vi "PID_old.vi"(6 "(t-1)in":dbl, 8 "error in":errorcluster, 9 "Low_Limit (0)":dbl, 10 "Up_Limit (40)":dbl, 11 "Ain":dbl=1.543879594670716 format="%0.2f") -> (0 "error out":errorcluster, 3 "Aout":dbl, 4 "(t-1)out":dbl)   [LabVIEW 2016]
doc: "Подпрограмма основана на непонятной\nмодели физического процесса и его\nреакции на ПИД регулирование.\nВ программу введена для сопоставления\nс предыдущими результатами."
panel:
  # "Подпрограмма основана на непонятной\nмодели физического процесса и его\nреакции на ПИД регулирование.\nВ программу введена для сопоставления\nс предыдущими результатами."
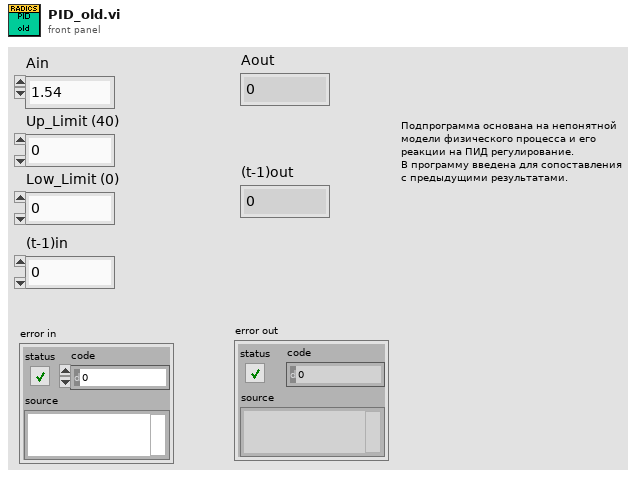
[diagram p1: front panel]
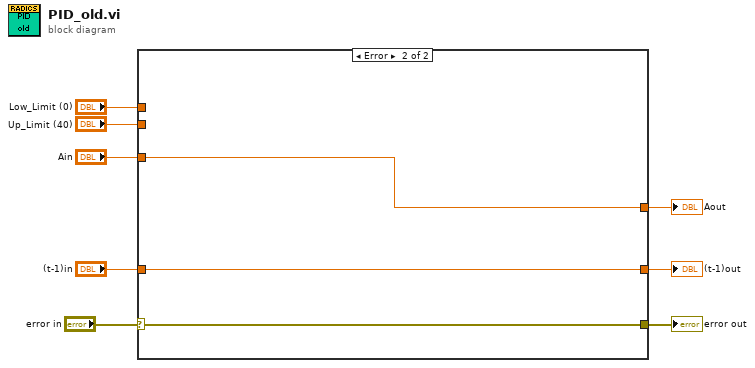
[diagram p0: block diagram]
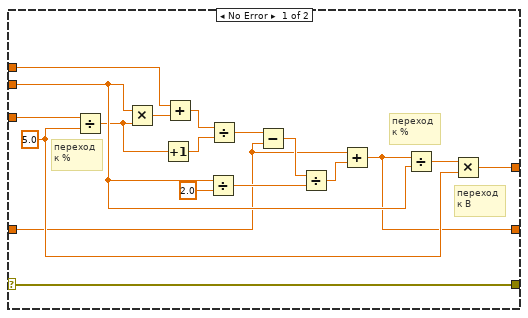
[diagram p2: hidden frame]
diagram:
  n1 = case shown="Error" "error in" {
    selector: "error in" -> [w11 w29]
    tunnel: [w26 w28] -> w8
    tunnel: "Up_Limit (40)" -> [w23 _]
    tunnel: "Low_Limit (0)" -> [w14 _]
    tunnel: "Ain" -> [w12 w28]
    tunnel: [w11 w29] -> w3
    tunnel: "(t-1)in" -> [w10 w27]
    tunnel: [w9 w27] -> w1
    frame No Error {
      w25 = 5.0 ("y")
      # "переход \nк В"
      # "переход \nк %"
      # "переход \nк %"
      n2 = Divide(x=w12, y=w25) -> (x/y=w15:dbl)
      n3 = Multiply(x=w23, y=w15) -> (x*y=w13:dbl)
      n4 = Increment(x=w15) -> (x+1=w17:dbl)
      n5 = Add(x=w14, y=w13) -> (x+y=w16:dbl)
      n6 = Divide(x=w23, y=2.0) -> (x/y=w21:dbl)
      n7 = Divide(x=w16, y=w17) -> (x/y=w18:dbl)
      n8 = Subtract(x=w18, y=w10) -> (x-y=w19:dbl)
      n9 = Divide(x=w19, y=w21) -> (x/y=w22:dbl)
      n10 = Add(x=w10, y=w22) -> (x+y=w9:dbl)
      n11 = Divide(x=w9, y=w23) -> (x/y=w24:dbl)
      n12 = Multiply(x=w24, y=w25) -> (x*y=w26:dbl)
    }
    frame Error {
    }
  }
  "Aout" <- w8
  "error out" <- w3
  "(t-1)out" <- w1
